vi "test_OneSessTwoPinOneSystemPinOneInstrOneSiteRes_CallGetConnFromPinsForAllDcPowerPinsOneSite_ReturnsTwoConn.vi"(8 "error in":errorcluster) -> (0 "error out":errorcluster, 2 "result":string, 3 "pass":bool)   [LabVIEW 2020, in "MeasurementServerTests.lvlib"]
uses:
  MeasurementServerTests.lvlib
  Runtime/MeasurementLink Session Management V1/Session Reservation/Connection with Session.ctl
  Runtime/MeasurementLink Session Management V1/Session Reservation/Connection.ctl
  Runtime/MeasurementLink niDCPower/Session Factory/Session Factory.lvclass
  D:/TAF/measurement-plugin-labview/Source/Runtime/MeasurementLink Instrument/ISession Factory/ISession Factory.lvclass
  Runtime/MeasurementLink Session Management V1/Session Reservation/Pin Type.ctl
  54d890a8-4121-421c-bfc5-08266fe71a04.vi
  777eb16d-c0be-4c50-a7a6-d4611c66469e.vi
  c3cb69a0-23cd-49fc-99d1-8c54773f0200.vi
  9ebf11f9-ce35-4e71-a0dd-d8a838d7b414.vi
  <vilib>/AdvancedString/1D String Array to Delimited String.vi
  9ebf11f9-ce35-4e71-a0dd-d8a838d7b414.vi/94283ac5-2298-4b3a-b57d-7be67da3787d.vi
  9ebf11f9-ce35-4e71-a0dd-d8a838d7b414.vi/f7d9c9cb-0251-4d67-81cb-70e1b0e8b69f.vi
  9ebf11f9-ce35-4e71-a0dd-d8a838d7b414.vi/48d9c053-c3ce-4ae4-8653-846fcb37df32.vi
  9ebf11f9-ce35-4e71-a0dd-d8a838d7b414.vi/38a8d12d-9165-42a0-bd04-ad62bed472d1.vi
  Runtime/MeasurementLink Session Management V1/Session Reservation/Get Connections Impl.vi
  <vilib>/JDP Science/JSONtext/Variant to JSON Text.vi
  <vilib>/JDP Science/JSONtext/LVClass Serializer/JSONtext LVClass Serializer.lvclass
  Runtime/MeasurementLink Session Management V1/Session Reservation/Session Reservation.lvclass
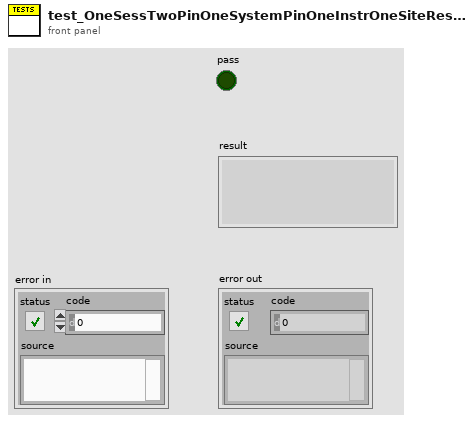
[diagram p1: front panel]
types:
  T1 = typedef "MeasurementLink Session Management V1.lvlib/Session Reservation.lvclass/Pin Type.ctl" = enum16{"DUT and System Pins", "System Pins"}
  T2 = typedef "MeasurementLink Session Management V1.lvlib/Session Reservation.lvclass/Connection.ctl" = cluster{"pin or relay name":string, "site":i32, "instrument type id":string, "channel":string}
  T3 = typedef "MeasurementLink Session Management V1.lvlib/Session Reservation.lvclass/Connection with Session.ctl" = cluster{"connection":T2, "session":variant}
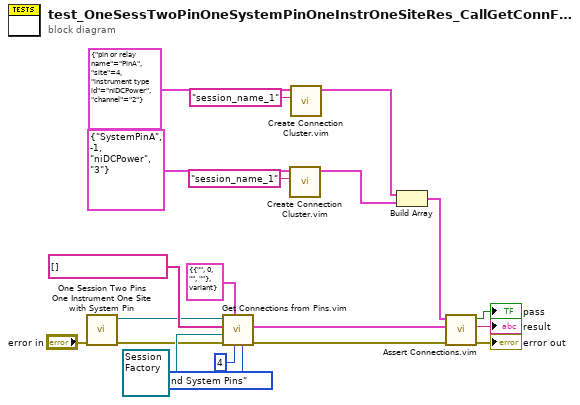
[diagram p0: block diagram]
diagram:
  n1 = call "One Session Two Pins One Instrument One Site with System Pin.vi"("error in"="error in") -> ("error out"=w3:errorcluster, "session reservation out"=w4:refnum<class "Session Reservation.lvclass">)  [unwired: 9 in]
  n2 = call "Get Connections from Pins.vim"("pin type"=Pin_Type."DUT and System Pins", "site"=4, "connection type"=T3 {"connection"={"pin or relay name"="", "site"=0, "instrument type id"="", "channel"=""}, "session"=variant} ("connection"), "error in"=w3, "session factory"=refnum<class "Session Factory.lvclass"> refnum ("MeasurementLink niDCPower.lvlib:Instrument.lvclass"), "pin or relay names"=string[] [], "session reservation in"=w4) -> ("error out"=w2:errorcluster, "connections"=w18:T3[])  [unwired: 2 in, 1 out]
  n3 = call "Create Connection Cluster.vim"("session in"="session_name_1", "hardware independent connection in"=T2 {"pin or relay name"="SystemPinA", "site"=-1, "instrument type id"="niDCPower", "channel"="3"} ("connection")) -> ("connection out"=w14:T3)  [unwired: 9 in]
  n4 = call "Create Connection Cluster.vim"("session in"="session_name_1", "hardware independent connection in"=T2 {"pin or relay name"="PinA", "site"=4, "instrument type id"="niDCPower", "channel"="2"} ("connection")) -> ("connection out"=w6:T3)  [unwired: 9 in]
  n5 = Build Array(w6, w14) -> (w13:T3[])
  n6 = call "Assert Connections.vim"("error in"=w2, "actual connections"=w18, "expected connections"=w13) -> ("error out"=→"error out":errorcluster, "result"=→"result":string, "pass"=→"pass":bool)  [unwired: 6 in]
